vi "Routing Templates Test Suite.vi"() -> ()   [LabVIEW 2020, in "Test_Routing Templates.lvlib"]
uses:
  Test_Routing Templates.lvlib
  <vilib>/addons/_JKI Toolkits/Caraya/classes/Test/Test.lvclass
panel:
  out "error out":errorcluster
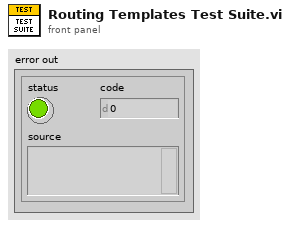
[diagram p1: front panel]
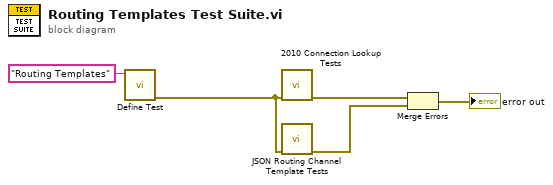
[diagram p0: block diagram]
diagram:
  n1 = call <vilib>:"Define Test.vi"("Label (VI Title)"="Routing Templates") -> ("error out"=w2:errorcluster)  [unwired: 10 in]
  n2 = call "2010 Connection Lookup Tests.vi"("error in"=w2) -> ("error out"=w5:errorcluster)  [unwired: 10 in]
  n3 = call "JSON Routing Channel Template Tests.vi"("error in"=w2) -> ("error out"=w1:errorcluster)  [unwired: 10 in]
  n4 = Merge Errors(w5, w1) -> (→"error out":errorcluster)
